vi "New Request.vi"(8 "error in (no error)":errorcluster, 9 "params":string, 10 "function":string, 11 "id":string) -> (0 "error out":errorcluster, 3 "request":refnum<class "request.lvclass">)   [LabVIEW 2015, in "request.lvclass"]
uses:
  request.lvclass
  request.lvclass/request.ctl
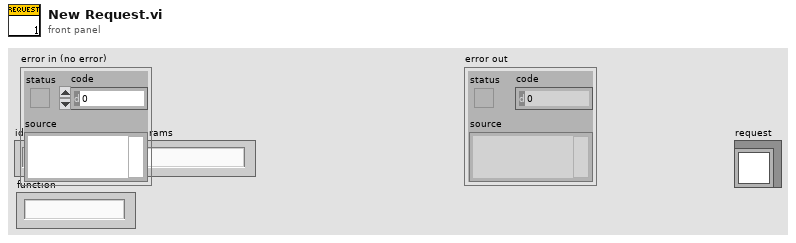
[diagram p1: front panel]
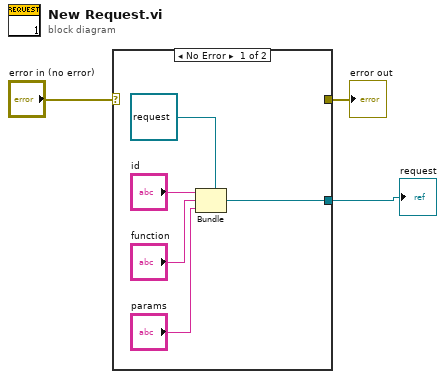
[diagram p0: block diagram]
diagram:
  n1 = case shown="No Error" "error in (no error)" {
    selector: "error in (no error)" -> [_ w9]
    tunnel: [_ w9] -> w2
    tunnel: [w4 _] -> w1
    frame No Error {
      n2 = Bundle(cluster=refnum<class "request.lvclass"> refnum ("request.lvclass"), "id", "function", "params") -> (w4:refnum<class "request.lvclass">)
    }
    frame Error {
    }
  }
  "error out" <- w2
  "request" <- w1
